vi "Frame control.vi"(10 "Getnext?":bool, 11 "frame":u8 format="%.0x") -> (2 "receivesequence":u8 format="%.0x", 3 "sendsequence":u8 format="%.0x")   [LabVIEW 2020]
uses:
  USB/KTC/Instrument/Electricity center/Electricity meter_DLMS/Subvi/DLL_Controlframe.dll
panel:
  out "return type":i32 format="%.0x"
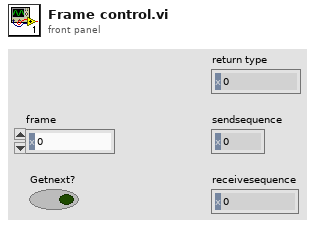
[diagram p1: front panel]
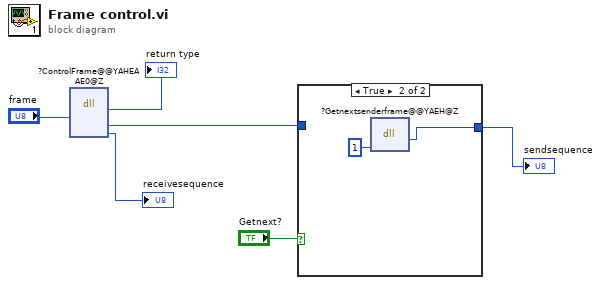
[diagram p0: block diagram]
diagram:
  n1 = dll-call lib="D:/USB/KTC/Instrument/Electricity center/Electricity meter_DLMS/Subvi/DLL_Controlframe.dll" fn="?ControlFrame@@YAHEAAE0@Z"("frame"="frame") -> ("return type"=→"return type":i32, "sendsequence"=w2:u8, "receivesequence"=→"receivesequence":u8)  [unwired: 6 in, 2 out]
  n2 = case shown="True" "Getnext?" {
    tunnel: w2 -> [w7 _]
    tunnel: [w7 w8] -> w1
    frame False {
    }
    frame True {
      n3 = dll-call lib="D:/USB/KTC/Instrument/Electricity center/Electricity meter_DLMS/Subvi/DLL_Controlframe.dll" fn="?Getnextsenderframe@@YAEH@Z"("true or false"=1) -> ("sendsequence"=w8:u8)  [unwired: 4 in, 2 out]
    }
  }
  "sendsequence" <- w1
